vi "总磷总氮启动参数对话框.vi"() -> (2 "确认":bool, 3 "元素":cluster{"命令":string, "data":variant})   [LabVIEW 2016, in "斯坦道通用流路CODmn.lvlib"]
panel:
  out "标液值":dbl caption="标液值："
  in  "取消":bool
  in  "确定":bool
  in  "量程切换":u16(ring)=2 items=["高量程", "低量程", "自动"]
  in  "站号":u16(ring)=1 items=["总氮"=2, "总磷"=1, "磷酸盐"=4]
  in  "控制命令":T1(ring)
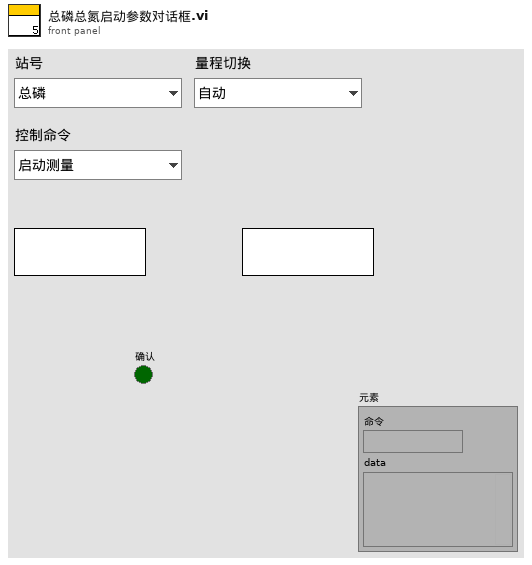
[diagram p1: front panel]
types:
  T1 = enum16{"启动测量", "标样核查", "零点核查", "跨度核查", "空白测试", "平行样测试", "加标回收", "空白校准", "标样校准", "初始化（清洗）", "停止测试", "仪器重启", "校时", "模式设置", "测量间隔设置"}
  T2 = typedef "LVStringsAndValuesArrayTypeDef_U16.ctl" = cluster{"String":string, "Value":u16}[]
  T3 = typedef "操作日志字段定义.ctl" = cluster{"时间":timestamp, "参数":string, "日志信息":string, "流程参数":string}
  T4 = cluster{"站号":u16, "量程切换":enum32{"H", "L", "AUTO"}, "控制命令":enum16{"启动测量", "标样核查", "零点核查", "跨度核查", "空白测试", "平行样测试", "加标回收", "空白校准", "标样校准", "初始化（清洗）", "停止测试", "仪器重启", "校时", "模式设置", "测量间隔设置", "盲样测试"}, "模式设置":enum16{"待机", "连续模式", "周期模式", "定点模式", "受控模式", "手动模式"}, "测量间隔":u16}
  T5 = cluster{"总磷跨度值":dbl, "总磷零点标准液浓度":dbl, "总磷跨度标准液浓度":dbl, "总磷标准液标准浓度":dbl, "总氮跨度值":dbl, "总氮零点标准液浓度":dbl, "总氮跨度标准液浓度":dbl, "总氮标准液标准浓度":dbl, "COD跨度值":dbl, "COD零点标准液浓度":dbl, "COD跨度标准液浓度":dbl, "COD标准液标准浓度":dbl, "氨氮跨度值":dbl, "氨氮零点标准液浓度":dbl, "氨氮跨度标准液浓度":dbl, "氨氮标准液标准浓度":dbl, "磷酸盐跨度值":dbl, "磷酸盐零点标准液浓度":dbl, "磷酸盐跨度标准液浓度":dbl, "磷酸盐标准液标准浓度":dbl, "硝氮跨度值":dbl, "硝氮零点标准液浓度":dbl, "硝氮跨度标准液浓度":dbl, "硝氮标准液标准浓度":dbl, "亚硝氮跨度值":dbl, "亚硝氮零点标准液浓度":dbl, "亚硝氮跨度标准液浓度":dbl, "亚硝氮标准液标准浓度":dbl, "硫化物跨度值":dbl, "硫化物零点标准液浓度":dbl, "硫化物跨度标准液浓度":dbl, "硫化物标准液标准浓度":dbl, "硅酸盐跨度值":dbl, "硅酸盐零点标准液浓度":dbl, "硅酸盐跨度标准液浓度":dbl, "硅酸盐标准液标准浓度":dbl, "总磷零点标准液偏差":dbl, "总磷跨度标准液偏差":dbl, "总磷标准液标准偏差":dbl, "总氮零点标准液偏差":dbl, "总氮跨度标准液偏差":dbl, "总氮标准液标准偏差":dbl, "COD零点标准液偏差":dbl, "COD跨度标准液偏差":dbl, "COD标准液标准偏差":dbl, "氨氮零点标准液偏差":dbl, "氨氮跨度标准液偏差":dbl, "氨氮标准液标准偏差":dbl, "磷酸盐零点标准液偏差":dbl, "磷酸盐跨度标准液偏差":dbl, "磷酸盐标准液标准偏差":dbl, "硝氮零点标准液偏差":dbl, "硝氮跨度标准液偏差":dbl, "硝氮标准液标准偏差":dbl, "亚硝氮零点标准液偏差":dbl, "亚硝氮跨度标准液偏差":dbl, "亚硝氮标准液标准偏差":dbl, "硫化物零点标准液偏差":dbl, "硫化物跨度标准液偏差":dbl, "硫化物标准液标准偏差":dbl, "硅酸盐零点标准液偏差":dbl, "硅酸盐跨度标准液偏差":dbl, "硅酸盐标准液标准偏差":dbl, "氟化物跨度值":dbl, "氟化物零点标准液浓度":dbl, "氟化物跨度标准液浓度":dbl, "氟化物标准液标准浓度":dbl, "氟化物零点标准液偏差":dbl, "氟化物跨度标准液偏差":dbl, "氟化物标准液标准偏差":dbl, "CODMn跨度值":dbl, "CODMn零点标准液浓度":dbl, "CODMn跨度标准液浓度":dbl, "CODMn标准液标准浓度":dbl, "CODMn零点标准液偏差":dbl, "CODMn跨度标准液偏差":dbl, "CODMn标准液标准偏差":dbl}
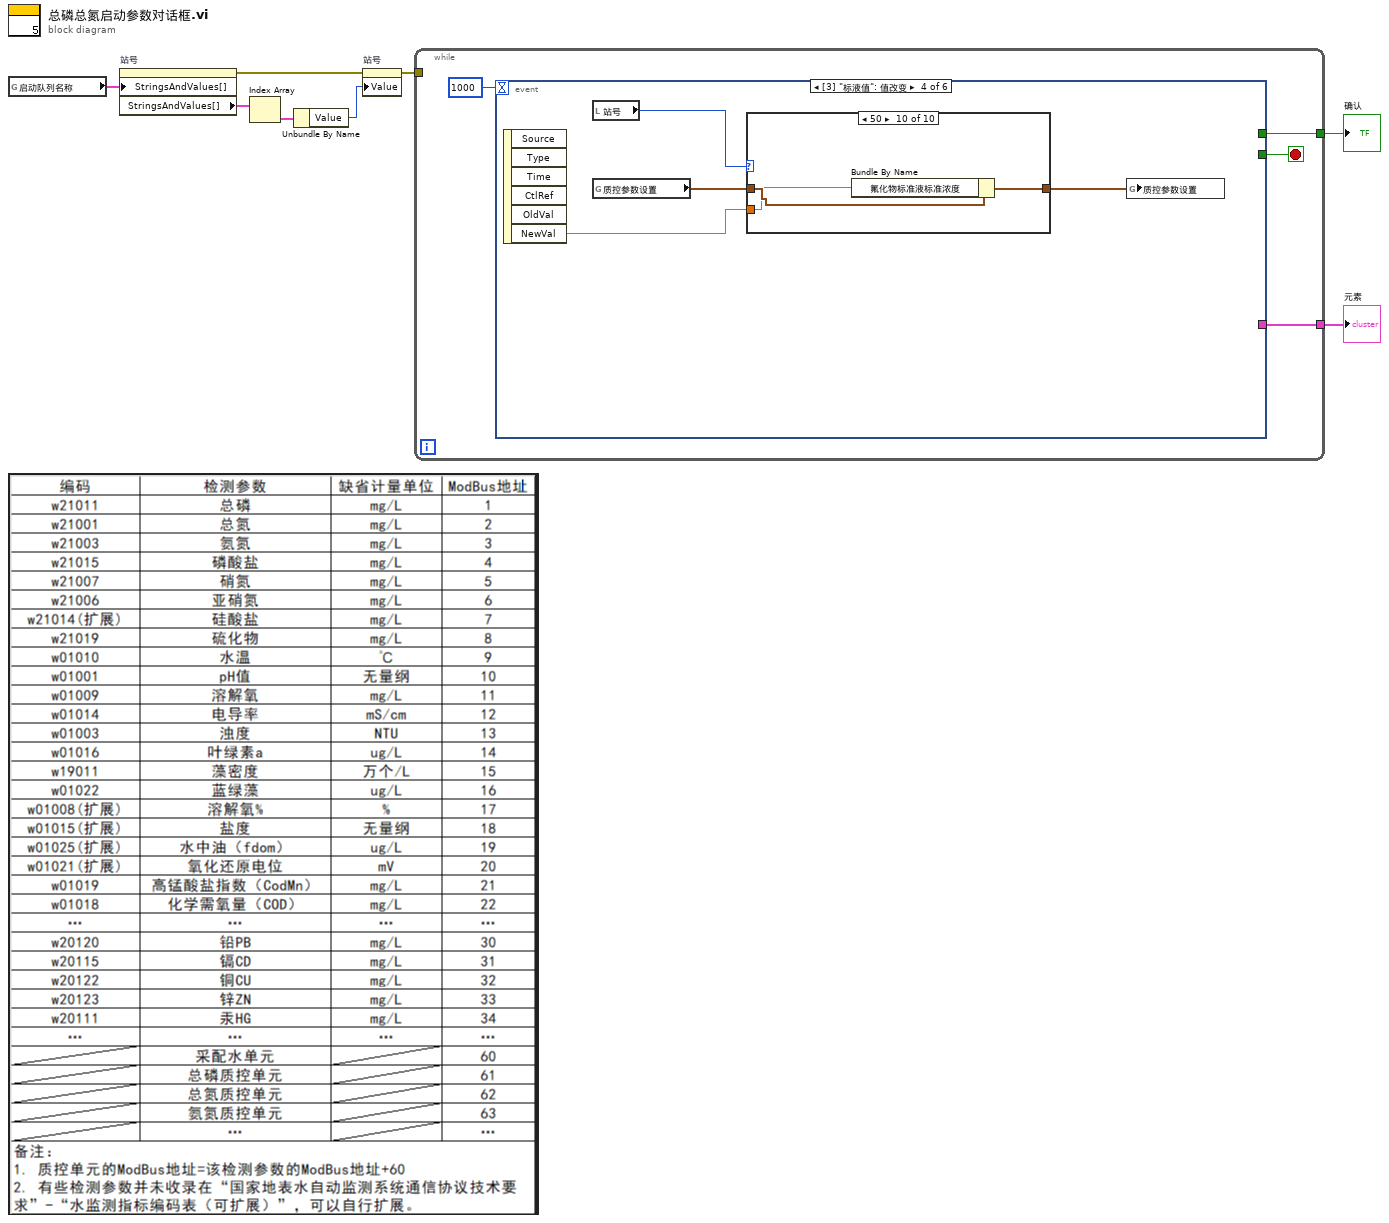
[diagram p0: block diagram]
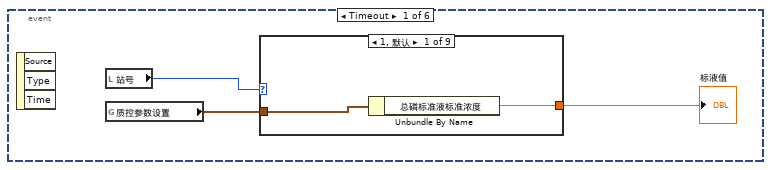
[diagram p2: hidden frame]
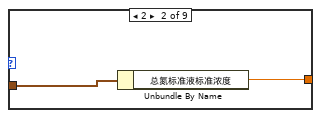
[diagram p3: hidden frame]
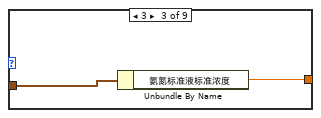
[diagram p4: hidden frame]
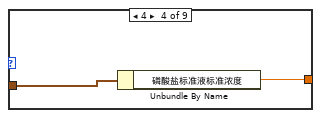
[diagram p5: hidden frame]
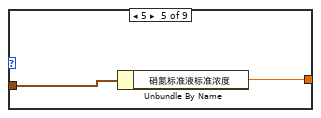
[diagram p6: hidden frame]
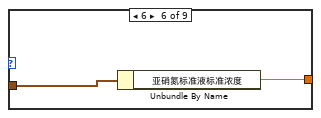
[diagram p7: hidden frame]
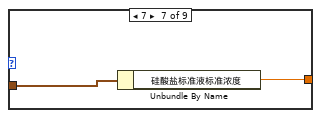
[diagram p8: hidden frame]
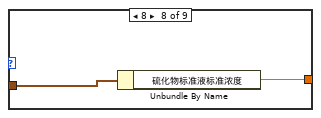
[diagram p9: hidden frame]
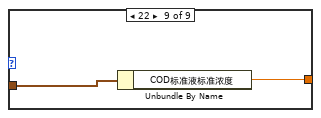
[diagram p10: hidden frame]
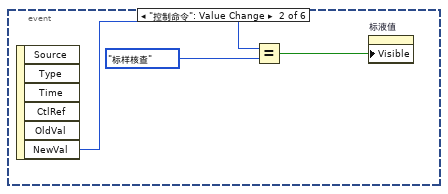
[diagram p11: hidden frame]
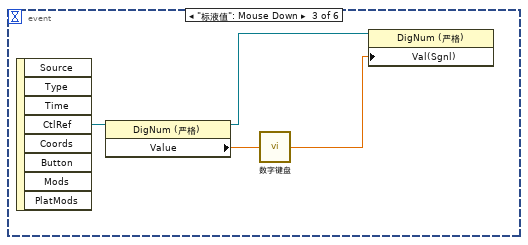
[diagram p12: hidden frame]
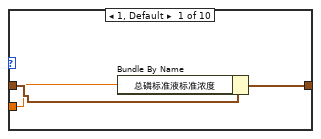
[diagram p13: hidden frame]
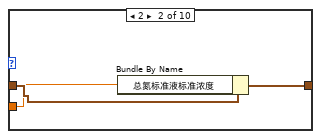
[diagram p14: hidden frame]
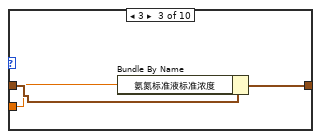
[diagram p15: hidden frame]
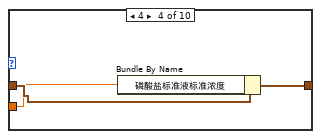
[diagram p16: hidden frame]
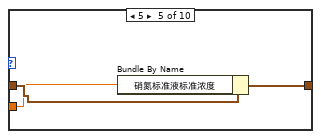
[diagram p17: hidden frame]
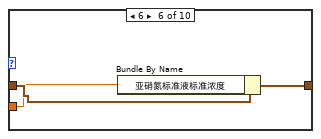
[diagram p18: hidden frame]
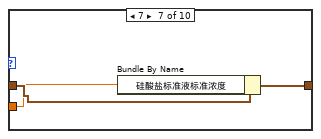
[diagram p19: hidden frame]
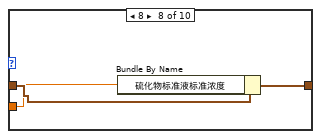
[diagram p20: hidden frame]
diagram:
  n1 = global read "model config var.vi" "启动队列名称"() -> (w6:cluster{"String":string, "Value":u16}[])
  n2 = property on="站号" class="Ring (严格)"("StringsAndValues[]"=w6) -> (error out=w5:errorcluster, "StringsAndValues[]"=w4:T2)  [unwired: 2 in, 1 out]
  n3 = Index Array(array=w4) -> (element=w3:cluster{"String":string, "Value":u16})  [unwired: 1 in]
  n4 = Unbundle By Name(w3) -> ("Value"=w2:u16)
  n5 = property on="站号" class="Ring (严格)"(error in=w5, "Value"=w2) -> (error out=w1:errorcluster)  [unwired: 1 in, 1 out]
  n6 = while {
    tunnel: [w10] -> w8
    tunnel: [w9] -> w7
    tunnel: w1 -> [_]
    stop <- w12 stop-if-true
    n7 = event shown="[3] \"标液值\": 值改变" {
      selector: _ -> [_ _ _ _ _ _]
      dyn-events: _ -> [_ _ _ _ _ _]
      timeout: 1000 -> [_ _ _ _ _ _]
      tunnel: [_ _ _ _ TRUE TRUE] -> w12
      tunnel: [_ _ _ _ TRUE _] -> w10
      tunnel: [_ _ _ _ w88 _] -> w9
      event Timeout {
        n8 = event-data() -> ()  [unwired: 1 in, 3 out]
        n9 = local read "站号"() -> (w14:u16)
        n10 = global read "总磷总氮断电保存全局变量.vi" "质控参数设置"() -> (w15:T5)
        n11 = case shown="1, 默认" w14 {
          tunnel: w15 -> [w17 w19 w21 w23 w25 w27 w29 w31 w33]
          tunnel: [w16 w18 w20 w22 w24 w26 w28 w30 w32] -> w13
          frame 1, Default {
            n12 = Unbundle By Name(w17) -> ("总磷标准液标准浓度"=w16:dbl)
          }
          frame 2 {
            n13 = Unbundle By Name(w19) -> ("总氮标准液标准浓度"=w18:dbl)
          }
          frame 3 {
            n14 = Unbundle By Name(w21) -> ("氨氮标准液标准浓度"=w20:dbl)
          }
          frame 4 {
            n15 = Unbundle By Name(w23) -> ("磷酸盐标准液标准浓度"=w22:dbl)
          }
          frame 5 {
            n16 = Unbundle By Name(w25) -> ("硝氮标准液标准浓度"=w24:dbl)
          }
          frame 6 {
            n17 = Unbundle By Name(w27) -> ("亚硝氮标准液标准浓度"=w26:dbl)
          }
          frame 7 {
            n18 = Unbundle By Name(w29) -> ("硅酸盐标准液标准浓度"=w28:dbl)
          }
          frame 8 {
            n19 = Unbundle By Name(w31) -> ("硫化物标准液标准浓度"=w30:dbl)
          }
          frame 22 {
            n20 = Unbundle By Name(w33) -> ("COD标准液标准浓度"=w32:dbl)
          }
        }
        "标液值" <- w13
      }
      event "控制命令": Value Change {
        n21 = event-data() -> ("NewVal"=w36:T1)  [unwired: 1 in, 5 out]
        n22 = Equal?(x=w36, y=T1."标样核查") -> (x = y?=w34:bool)
        n23 = property on="标液值" class="DigNum (严格)"("Visible"=w34) -> ()  [unwired: 2 in, 2 out]
      }
      event "标液值": Mouse Down {
        n24 = event-data() -> ("CtlRef"=w40:refnum<vi>)  [unwired: 1 in, 7 out]
        n25 = property class="DigNum (严格)"(reference=w40) -> (reference out=w37:refnum<vi>, "Value"=w39:dbl)  [unwired: 1 in, 1 out]
        n26 = call "数字键盘.vi"("OldNumber"=w39) -> ("NewNumber"=w38:dbl)
        n27 = property class="DigNum (严格)"(reference=w37, "Val(Sgnl)"=w38) -> ()  [unwired: 1 in, 2 out]
      }
      event "标液值": Value Change {
        n28 = event-data() -> ("NewVal"=w42:dbl)  [unwired: 1 in, 5 out]
        n29 = local read "站号"() -> (w44:u16)
        n30 = global read "总磷总氮断电保存全局变量.vi" "质控参数设置"() -> (w43:T5)
        n31 = case shown="50" w44 {
          tunnel: w43 -> [w47 w50 w53 w56 w59 w62 w65 w68 w71 w74]
          tunnel: [w45 w48 w51 w54 w57 w60 w63 w66 w69 w72] -> w41
          tunnel: w42 -> [w46 w49 w52 w55 w58 w61 w64 w67 w70 w73]
          frame 1, Default {
            n32 = Bundle By Name(cluster=w47, "总磷标准液标准浓度"=w46) -> (w45:T5)
          }
          frame 2 {
            n33 = Bundle By Name(cluster=w50, "总氮标准液标准浓度"=w49) -> (w48:T5)
          }
          frame 3 {
            n34 = Bundle By Name(cluster=w53, "氨氮标准液标准浓度"=w52) -> (w51:T5)
          }
          frame 4 {
            n35 = Bundle By Name(cluster=w56, "磷酸盐标准液标准浓度"=w55) -> (w54:T5)
          }
          frame 5 {
            n36 = Bundle By Name(cluster=w59, "硝氮标准液标准浓度"=w58) -> (w57:T5)
          }
          frame 6 {
            n37 = Bundle By Name(cluster=w62, "亚硝氮标准液标准浓度"=w61) -> (w60:T5)
          }
          frame 7 {
            n38 = Bundle By Name(cluster=w65, "硅酸盐标准液标准浓度"=w64) -> (w63:T5)
          }
          frame 8 {
            n39 = Bundle By Name(cluster=w68, "硫化物标准液标准浓度"=w67) -> (w66:T5)
          }
          frame 22 {
            n40 = Bundle By Name(cluster=w71, "COD标准液标准浓度"=w70) -> (w69:T5)
          }
          frame 50 {
            n41 = Bundle By Name(cluster=w74, "氟化物标准液标准浓度"=w73) -> (w72:T5)
          }
        }
        n42 = global write "总磷总氮断电保存全局变量.vi" "质控参数设置"(w41) -> ()
      }
      event "确定": Value Change {
        n43 = event-data() -> ()  [unwired: 1 in, 6 out]
        n44 = call <vilib>:"Space Constant.vi"() -> ("String"=w78:string)
        n45 = property on="控制命令" class="Enum (严格)"() -> ("RingText.Text"=w79:string)  [unwired: 2 in, 2 out]
        n46 = Concatenate Strings("手动启动" ("日志信息"), w78, w79) -> (w75:string)
        n47 = Get Date/Time In Seconds() -> (seconds since 1Jan1904=w80:timestamp)
        n48 = property on="站号" class="Ring (严格)"() -> ("RingText.Text"=w77:string)  [unwired: 2 in, 2 out]
        n49 = Bundle By Name(cluster=T4 {"站号"=1, "量程切换"=enum."AUTO", "控制命令"=enum."启动测量", "模式设置"=enum."待机", "测量间隔"=0} ("参数"), "站号"="站号", "量程切换"="量程切换", "控制命令"="控制命令") -> (w86:T4)
        n50 = Bundle By Name(cluster=T3 {"时间"=timestamp(0 s since 1904-01-01), "参数"="", "日志信息"="", "流程参数"=""} ("data in"), "时间"=w80, "参数"=w77, "日志信息"=w75) -> (w81:T3)
        n51 = call "总磷总氮启动命令.vi"("参数"=w86) -> ("启动命令"=w88:cluster{"命令":string, "data":variant})  [unwired: 10 in]
        n52 = call "总磷总氮操作日志.vi"("data in"=w81) -> ()  [unwired: 10 in, 1 out]
      }
      event "取消": Value Change; Panel Close {
        n53 = event-data() -> ()  [unwired: 1 in, 3 out]
      }
    }
  }
  "元素" <- w7
  "确认" <- w8
